vi "get desired keys.vi"(8 "error in":errorcluster, 11 "Custom Controller Module configuration in":refnum<class "Custom Controller Module configuration.lvclass">) -> (0 "error out":errorcluster, 2 "desired keys":string[](array[string]), 3 "Custom Controller Module configuration out":refnum<class "Custom Controller Module configuration.lvclass">)   [LabVIEW 2013, in "Custom Controller Module configuration.lvclass"]
uses:
  Custom Controller Module configuration.lvclass
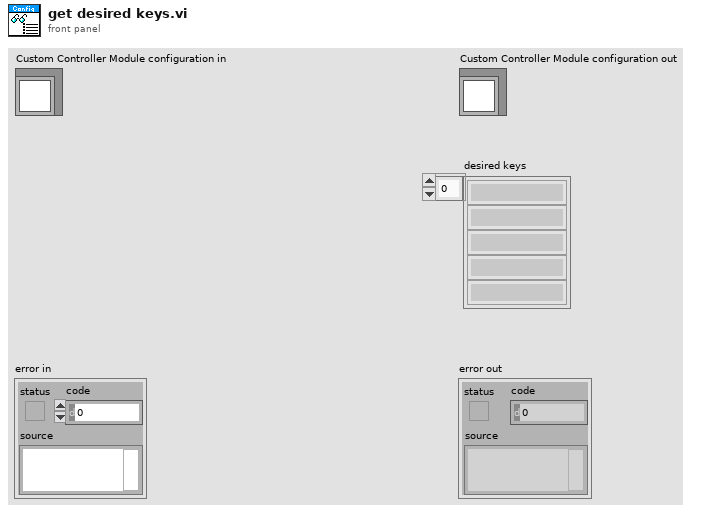
[diagram p1: front panel]
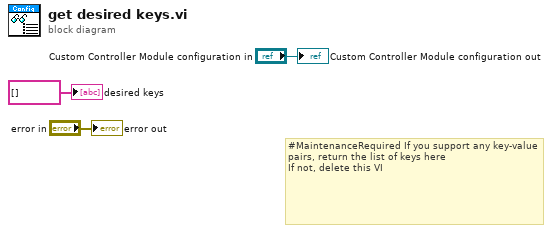
[diagram p0: block diagram]
diagram:
  # "#MaintenanceRequired If you support any key-value pairs, return the list of keys here\nIf not, delete this VI"
  "error out" <- "error in"
  "Custom Controller Module configuration out" <- "Custom Controller Module configuration in"
  "desired keys" <- string[] [] ("desired keys")
